vi "Get Local Error Manager Name.vi"() -> (0 "Error Manager ID":string)   [LabVIEW 2026, in "TALOS.lvlib"]
uses:
  TALOS.lvlib
  Global Memory.vi
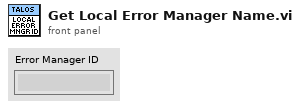
[diagram p1: front panel]
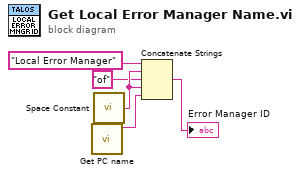
[diagram p0: block diagram]
diagram:
  n1 = call "Get PC name.vi"() -> ("Hostname"=w1:string)  [unwired: 10 in, 1 out]
  n2 = call <vilib>:"Space Constant.vi"() -> ("String"=w4:string)
  n3 = Concatenate Strings("Local Error Manager" ("uService ID"), w4, "of" ("string"), w4, w1) -> (→"Error Manager ID":string)
